vi "Format File Header.vi"(5 "Header Data (Empty)":string[](array[string]), 7 "Header Titles (Empty)":string[](array[string]), 8 "Error In":errorcluster) -> (0 "Error Out":errorcluster, 3 "File Header":string)   [LabVIEW 2012]
doc: "Creates the file headers for the log file."
uses:
  <vilib>/ErrorRing/Error Ring.xnode
  <vilib>/Utility/error.llb/Error Cluster From Error Code.vi
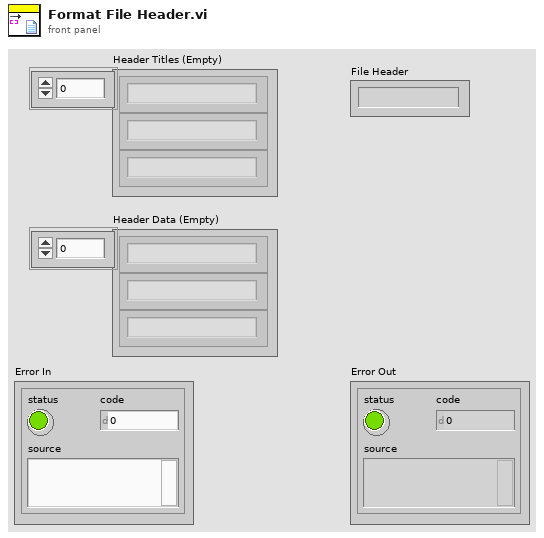
[diagram p1: front panel]
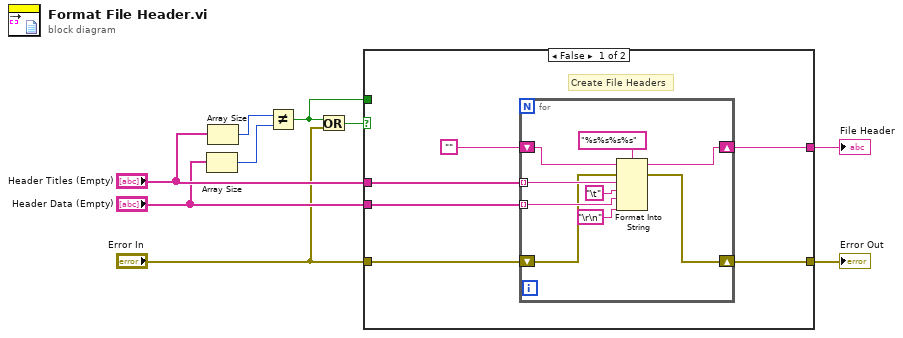
[diagram p0: block diagram]
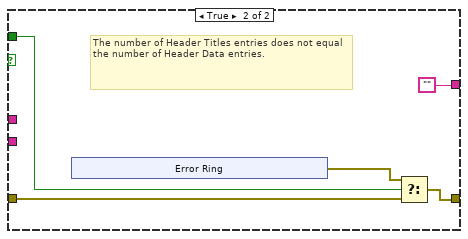
[diagram p2: hidden frame]
diagram:
  n1 = Array Size(array="Header Data (Empty)") -> (size(s)=w5:i32)
  n2 = Array Size(array="Header Titles (Empty)") -> (size(s)=w6:i32)
  n3 = Not Equal?(x=w6, y=w5) -> (x != y?=w2:bool)
  n4 = Or(x=w2, y="Error In") -> (x .or. y?=w4:bool)
  n5 = case shown="False" w4 {
    tunnel: [w10 w26] -> w9
    tunnel: "Header Titles (Empty)" -> [w15 _]
    tunnel: "Header Data (Empty)" -> [w14 _]
    tunnel: "Error In" -> [w11 w27]
    tunnel: w2 -> [_ w28]
    tunnel: [w12 ""] -> w1
    frame False {
      # "Create File Headers"
      n6 = for {
        tunnel: w15 -> [w20] mode=indexing
        tunnel: w14 -> [w19] mode=indexing
        shift-right: [w18] -> w12
        shift-left: "" -> [w21]
        shift-right: [w16] -> w10
        shift-left: w11 -> [w17]
        n7 = Format Into String(format string="%s%s%s%s", initial string=w21, error in=w17, w20, "\t", w19, "\r\n") -> (resulting string=w18:string, error out=w16:errorcluster)
      }
    }
    frame True {
      # "The number of Header Titles entries does not equal the number of Header Data entries."
      n8 = xnode "Error Ring"() -> ("error out"=w25:errorcluster)
      n9 = Select(t=w25, s=w28, f=w27) -> (s? t:f=w26:errorcluster)
    }
  }
  "Error Out" <- w9
  "File Header" <- w1
